vi "Uninit.vi"(11 "UI in":refnum<class "UI.lvclass">) -> (3 "UI out":refnum<class "UI.lvclass">)   [LabVIEW 2020, in "UI.lvlib" / "UI.lvclass"]
doc: "This method is the inverse of the Pre Launch Init.vi. This method is called unconditionally at the end of an actor's lifetime, even if there was an error in Pre Launch Init.vi. Note that the self Enqueuer for the actor is already invalid by the time this VI executes: within this method, the actor may send messages to its caller but not to itself. This method executes before Last Ack is sent.\n\nThis method neither receives nor produces an error cluster. It is designed to provide an unconditional release of acquired resources. Any error raised during release is considered to be irrelevant to the actor's lifetime. If the actor truly needs to report some error status, it may send a message to caller or include information within itself that callers can examine when handling Last Ack."
uses:
  UI.lvclass
  UI.lvclass/UI.ctl
  <vilib>/ActorFramework/Actor/Actor.lvclass
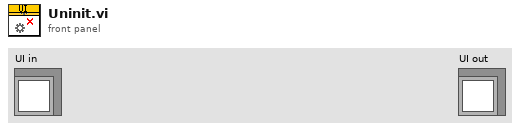
[diagram p1: front panel]
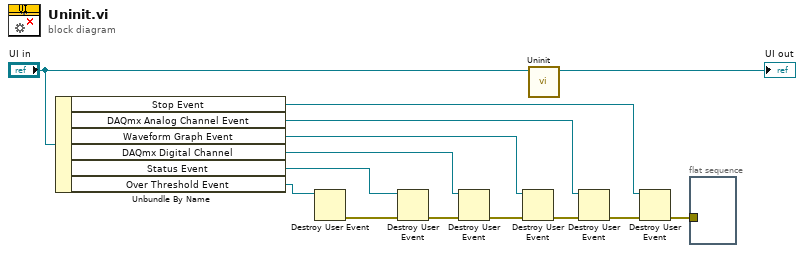
[diagram p0: block diagram]
diagram:
  n1 = Unbundle By Name("UI in") -> ("Stop Event"=w4:refnum<user-event>, "DAQmx Analog Channel Event"=w7:refnum<user-event>, "Waveform Graph Event"=w8:refnum<user-event>, "DAQmx Digital Channel"=w11:refnum<user-event>, "Status Event"=w12:refnum<user-event>, "Over Threshold Event"=w2:refnum<user-event>)
  n2 = Destroy User Event(user event=w2) -> (error out=w1:errorcluster)  [unwired: 1 in]
  n3 = Destroy User Event(user event=w12, error in=w1) -> (error out=w10:errorcluster)
  n4 = Destroy User Event(user event=w11, error in=w10) -> (error out=w9:errorcluster)
  n5 = Destroy User Event(user event=w8, error in=w9) -> (error out=w6:errorcluster)
  n6 = call-parent "Uninit.vi"("Actor in"="UI in") -> ("Actor out"=→"UI out":refnum<class "UI.lvclass">)  [unwired: 10 in]
  n7 = Destroy User Event(user event=w7, error in=w6) -> (error out=w5:errorcluster)
  n8 = Destroy User Event(user event=w4, error in=w5) -> (error out=w3:errorcluster)
  n9 = flat-sequence {
    tunnel: w3 -> [_]
    frame #0 {
    }
  }
